vi "macro_Apply_Deadband.vi"   [LabVIEW 2019, in "Trajectory_Library.lvlib"]
uses:
  Trajectory_Library.lvlib
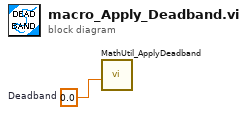
[diagram p0: block diagram]
diagram:
  w1 = 0.0  # Deadband
  n1 = call "MathUtil_ApplyDeadband.vi"("Deadband"=w1) -> ()  [unwired: 10 in, 1 out]
